vi "CreateInitialValueAtRegister.vi"(0 "JSON":string, 1 "Register Index":u32, 2 "Value":variant, 3 "DataType":string, 5 "error in (no error)":errorcluster) -> (14 "<JSON>":string caption="<JSON>Merged", 19 "error out":errorcluster)   [LabVIEW 2017]
uses:
  <vilib>/JDP Science/JSONtext/JSONtext.lvlib
  94c79dad-4e9f-4eed-9efb-c605e2042fdb.vi
  eabd0766-5937-45a3-a5b9-4c662874f0da.vi
  00b83709-2709-403f-811c-68af91155cf1.vi
  57c48c52-2b49-40e4-92c0-ad1d79bdde24.vi
  dd63b98d-9a67-4c1d-adda-15964cb9bf70.vi
  2c5920fd-cee7-4d25-abda-fef0a3110257.vi
  0fb49ede-86d8-496f-be7e-d7222a0d96bc.vi
  66e77878-1ad1-4d56-98dc-5196c7a0bcf4.vi
  bb7847d8-7d19-4bb0-8e5a-ad9ccdb5d84f.vi
  91abbd68-445d-4aa2-a4b3-1b04da193de2.vi
  9bc7ad0a-bdeb-4c04-80fd-e4274a378abd.vi
  8ec20e0a-0c61-4861-829d-d421042543f2.vi
  1d32db34-b911-4283-954b-5abf14300159.vi
  95dec7b1-d680-4a39-a329-a6123795ff0d.vi
  8d203c44-1999-4304-8263-79fa894e32f6.vi
  e51c4e9c-d1b6-4e11-aa13-962035e5aeed.vi
  <vilib>/Utility/Data Type/NI_Data Type.lvlib
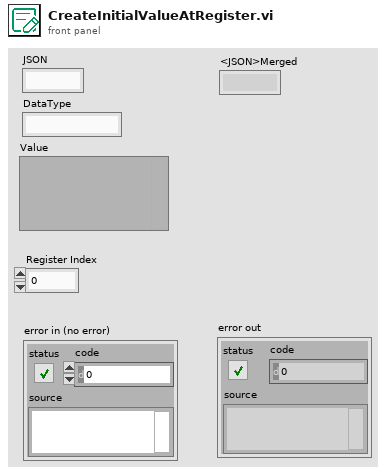
[diagram p1: front panel]
types:
  T1 = typedef "NI_Data Type.lvlib/Data Type.ctl" = enum8{"Invalid Type", "Void", "I8", "I16", "I32", "I64", "U8", "U16", "U32", "U64", "Single Float", "Double Float", "Extended Float", "Single Complex", "Double Complex", "Extended Complex", "Enum U8", "Enum U16", "Enum U32", "Enum U64", "Single Float With Unit", "Double Float With Unit", "Extended Float With Unit", "Single Complex with Unit", "Double Complex with Unit", "Extended Complex with Unit", "Boolean", "String", "Path", "Picture", "Tag", "Array", "Cluster", "Variant", "LV Variant", "Waveform", "Timestamp", "Digital Waveform", "Digital Data", "ExpressData", "Refnum", "External Data", "VI", "Poly VI", "LabVIEW Class Instance", "Fixed Point"}
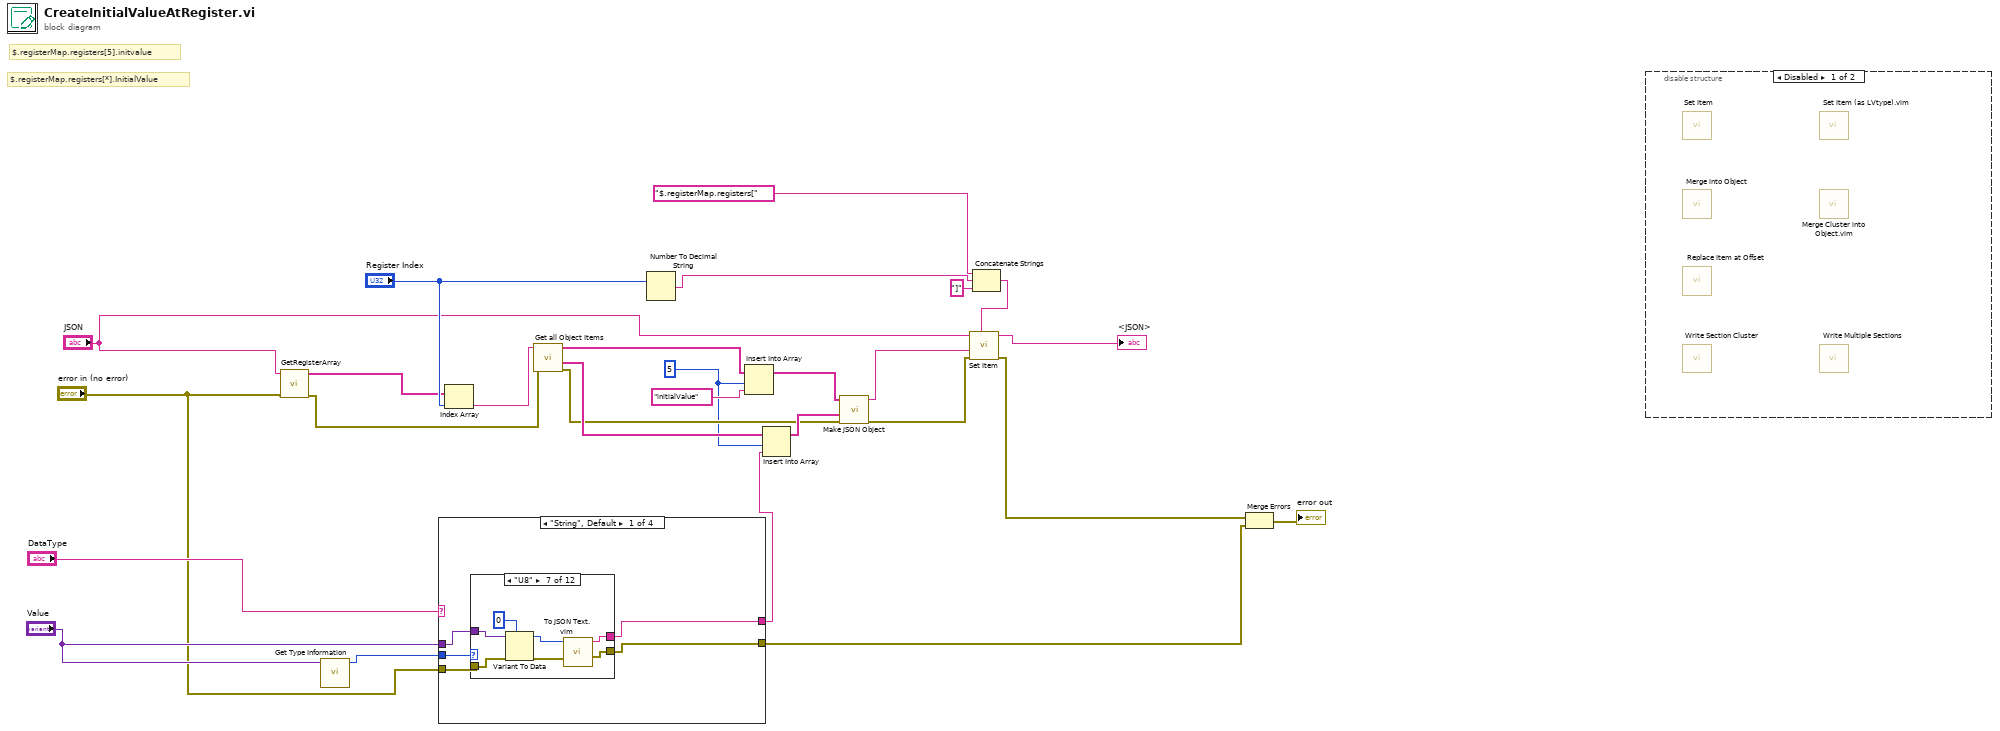
[diagram p0: block diagram]
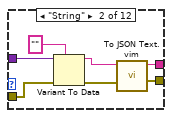
[diagram p3: hidden frame]
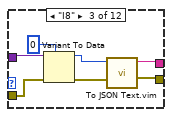
[diagram p4: hidden frame]
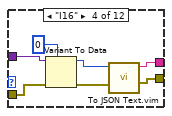
[diagram p5: hidden frame]
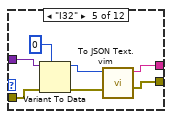
[diagram p6: hidden frame]
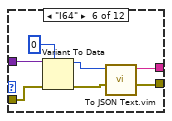
[diagram p7: hidden frame]
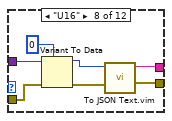
[diagram p8: hidden frame]
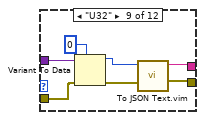
[diagram p9: hidden frame]
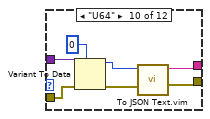
[diagram p10: hidden frame]
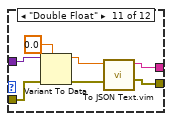
[diagram p11: hidden frame]
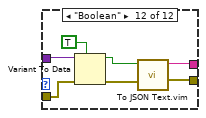
[diagram p12: hidden frame]
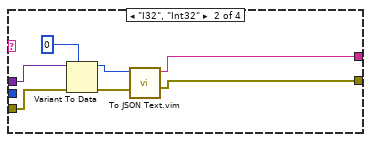
[diagram p13: hidden frame]
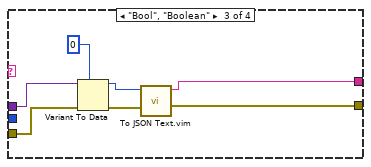
[diagram p14: hidden frame]
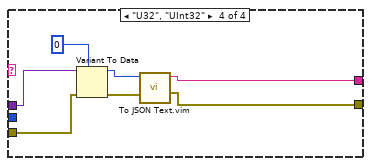
[diagram p15: hidden frame]
diagram:
  w17 = 5 ("index")
  # "$.registerMap.registers[*].InitialValue"
  # "$.registerMap.registers[5].initvalue"
  n1 = call "GetRegisterArray.vi"("error in (no error)"="error in (no error)", "JSON Text"="JSON") -> ("error out"=w2:errorcluster, "Register Array"=w1:string[])  [unwired: 8 in]
  n2 = call <vilib>:"Get Type Information.vi"("Variant"="Value") -> ("Type"=w12:T1)  [unwired: 6 in, 4 out]
  n3 = case shown="\"String\", Default" "DataType" {
    tunnel: "Value" -> [w32 w114 w124 w131]
    tunnel: [w29 w115 w121 w128] -> w9
    tunnel: w12 -> [w31 _ _ _]
    tunnel: "error in (no error)" -> [w30 w113 w120 w127]
    tunnel: [w28 w111 w118 w125] -> w7
    frame "String", Default {
      n4 = case shown="\"U8\"" w31 {
        tunnel: w32 -> [_ w40 w46 w53 w60 w67 w74 w81 w88 w95 w102 w108]
        tunnel: [_ w37 w44 w52 w58 w66 w72 w79 w86 w93 w100 w107] -> w29
        tunnel: w30 -> [w33 w36 w43 w50 w57 w64 w71 w78 w85 w92 w99 w106]
        tunnel: [w33 w34 w41 w48 w55 w62 w69 w76 w83 w90 w97 w104] -> w28
        frame "Invalid Type", Default {
        }
        frame "String" {
          n5 = Variant To Data(error in=w36, type="", Variant=w40) -> (data=w38:string, error out=w35:errorcluster)
          n6 = call "To JSON Text.vim"("error in (no error)"=w35, "Anything"=w38) -> ("error out"=w34:errorcluster, "<JSON>"=w37:string)  [unwired: 8 in]
        }
        frame "I8" {
          n7 = Variant To Data(error in=w43, type=i8 0, Variant=w46) -> (data=w47:i8, error out=w42:errorcluster)
          n8 = call "To JSON Text.vim"("error in (no error)"=w42, "Anything"=w47) -> ("error out"=w41:errorcluster, "<JSON>"=w44:string)  [unwired: 8 in]
        }
        frame "I16" {
          n9 = Variant To Data(error in=w50, type=i16 0, Variant=w53) -> (data=w54:i16, error out=w49:errorcluster)
          n10 = call "To JSON Text.vim"("error in (no error)"=w49, "Anything"=w54) -> ("error out"=w48:errorcluster, "<JSON>"=w52:string)  [unwired: 8 in]
        }
        frame "I32" {
          n11 = Variant To Data(error in=w57, type=0, Variant=w60) -> (data=w61:i32, error out=w56:errorcluster)
          n12 = call "To JSON Text.vim"("error in (no error)"=w56, "Anything"=w61) -> ("error out"=w55:errorcluster, "<JSON>"=w58:string)  [unwired: 8 in]
        }
        frame "I64" {
          n13 = Variant To Data(error in=w64, type=i64 0, Variant=w67) -> (data=w68:i64, error out=w63:errorcluster)
          n14 = call "To JSON Text.vim"("error in (no error)"=w63, "Anything"=w68) -> ("error out"=w62:errorcluster, "<JSON>"=w66:string)  [unwired: 8 in]
        }
        frame "U8" {
          n15 = Variant To Data(error in=w71, type=u8 0, Variant=w74) -> (data=w75:u8, error out=w70:errorcluster)
          n16 = call "To JSON Text.vim"("error in (no error)"=w70, "Anything"=w75) -> ("error out"=w69:errorcluster, "<JSON>"=w72:string)  [unwired: 8 in]
        }
        frame "U16" {
          n17 = Variant To Data(error in=w78, type=u16 0, Variant=w81) -> (data=w82:u16, error out=w77:errorcluster)
          n18 = call "To JSON Text.vim"("error in (no error)"=w77, "Anything"=w82) -> ("error out"=w76:errorcluster, "<JSON>"=w79:string)  [unwired: 8 in]
        }
        frame "U32" {
          n19 = Variant To Data(error in=w85, type=u32 0, Variant=w88) -> (data=w89:u32, error out=w84:errorcluster)
          n20 = call "To JSON Text.vim"("error in (no error)"=w84, "Anything"=w89) -> ("error out"=w83:errorcluster, "<JSON>"=w86:string)  [unwired: 8 in]
        }
        frame "U64" {
          n21 = Variant To Data(error in=w92, type=u64 0, Variant=w95) -> (data=w96:u64, error out=w91:errorcluster)
          n22 = call "To JSON Text.vim"("error in (no error)"=w91, "Anything"=w96) -> ("error out"=w90:errorcluster, "<JSON>"=w93:string)  [unwired: 8 in]
        }
        frame "Double Float" {
          n23 = Variant To Data(error in=w99, type=0.0, Variant=w102) -> (data=w103:dbl, error out=w98:errorcluster)
          n24 = call "To JSON Text.vim"("error in (no error)"=w98, "Anything"=w103) -> ("error out"=w97:errorcluster, "<JSON>"=w100:string)  [unwired: 8 in]
        }
        frame "Boolean" {
          n25 = Variant To Data(error in=w106, type=TRUE, Variant=w108) -> (data=w110:bool, error out=w105:errorcluster)
          n26 = call "To JSON Text.vim"("error in (no error)"=w105, "Anything"=w110) -> ("error out"=w104:errorcluster, "<JSON>"=w107:string)  [unwired: 8 in]
        }
      }
    }
    frame "I32", "Int32" {
      n27 = Variant To Data(error in=w113, type=0, Variant=w114) -> (data=w116:i32, error out=w112:errorcluster)
      n28 = call "To JSON Text.vim"("error in (no error)"=w112, "Anything"=w116) -> ("error out"=w111:errorcluster, "<JSON>"=w115:string)  [unwired: 8 in]
    }
    frame "Bool", "Boolean" {
      n29 = Variant To Data(error in=w120, type=u16 0, Variant=w124) -> (data=w122:u16, error out=w119:errorcluster)
      n30 = call "To JSON Text.vim"("error in (no error)"=w119, "Anything"=w122) -> ("error out"=w118:errorcluster, "<JSON>"=w121:string)  [unwired: 8 in]
    }
    frame "U32", "UInt32" {
      n31 = Variant To Data(error in=w127, type=u32 0, Variant=w131) -> (data=w129:u32, error out=w126:errorcluster)
      n32 = call "To JSON Text.vim"("error in (no error)"=w126, "Anything"=w129) -> ("error out"=w125:errorcluster, "<JSON>"=w128:string)  [unwired: 8 in]
    }
  }
  n33 = Index Array(array=w1, index="Register Index") -> (element=w26:string)
  n34 = call <vilib>:"Get all Object Items.vi"("error in (no error)"=w2, "JSON"=w26) -> ("error out"=w18:errorcluster, "<JSON>"=w23:string[], "Item Names"=w25:string[])  [unwired: 6 in, 1 out]
  n35 = Number To Decimal String(number="Register Index") -> (decimal integer string=w15:string)  [unwired: 1 in]
  n36 = Insert Into Array(array=w25, index=w17, new element="initialValue") -> (w22:string[])
  n37 = Insert Into Array(array=w23, index=w17, new element=w9) -> (w21:string[])
  n38 = call <vilib>:"Make JSON Object.vi"("error in (no error)"=w18, "JSON Items"=w21, "Item Names"=w22) -> ("error out"=w6:errorcluster, "<JSON>"=w20:string)  [unwired: 7 in]
  n39 = Concatenate Strings("$.registerMap.registers[" ("$Path or Item Name"), w15, "]" ("string")) -> (w10:string)
  n40 = call <vilib>:"Set Item.vi"("$Path or Item Name"=w10, "error in (no error)"=w6, "JSON to Insert"=w20, "JSON"="JSON") -> ("error out"=w5:errorcluster, "<JSON>"=→"<JSON>":string)  [unwired: 4 in, 1 out]
  n41 = Merge Errors(w5, w7) -> (→"error out":errorcluster)
  n42 = disable-structure shown="Disabled" {
    frame Disabled {
      n43 = call <vilib>:"Set Item.vi"() -> ()  [unwired: 8 in, 3 out]
      n44 = call <vilib>:"Merge into Object.vi"() -> ()  [unwired: 9 in, 2 out]
      n45 = call <vilib>:"Replace Item at Offset.vi"() -> ()  [unwired: 10 in, 2 out]
      n46 = call <vilib>:"Write Section Cluster.vi"() -> ()  [unwired: 9 in, 2 out]
      n47 = call "Set Item (as LVtype).vim"() -> ()  [unwired: 8 in, 3 out]
      n48 = call "Merge Cluster into Object.vim"() -> ()  [unwired: 9 in, 2 out]
      n49 = call <vilib>:"Write Multiple Sections.vi"() -> ()  [unwired: 9 in, 2 out]
    }
    frame Enabled {
    }
  }
